vi "Read All Segments.vi"(8 "error in (no error)":errorcluster, 9 "Timeout (10000 ms)":u32=10000, 10 "Source (0: Channel 1)":u16(ring) items=["Channel 1", "Channel 2", "Channel 3", "Channel 4", "Memory 1", "Memory 2", "Memory 3", "Memory 4", "Function 1", "Function 2", "Function 3", "Function 4", "Function 5", "Function 6", "Function 7", "Function 8"], 11 "VISA resource name":refnum<visa-resource-name>) -> (0 "error out":errorcluster, 2 "Max Waveform":waveform(dbl)[](graph), 3 "VISA resource name out":refnum<visa-resource-name>)   [LabVIEW 2013, in "LeCroy Wave Series.lvlib"]
doc: "Returns the alls segments of waveform the oscilloscope acquired for the specified channel. The waveform is from an acquisition that you initiate prior to calling this VI.\n\nNote:\n\nSequence Acquisitions are not supported by WaveSurfer models."
uses:
  LeCroy Wave Series.lvlib
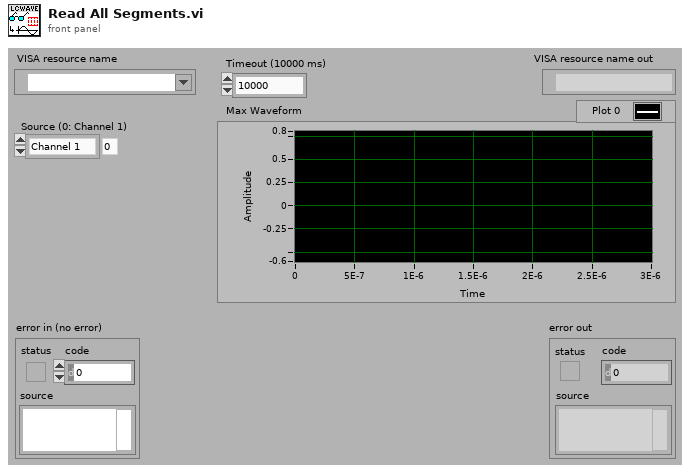
[diagram p1: front panel]
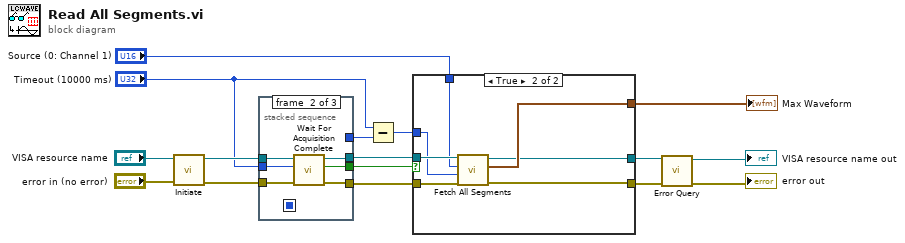
[diagram p0: block diagram]
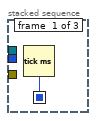
[diagram p2: hidden frame]
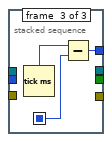
[diagram p3: hidden frame]
diagram:
  n1 = call "Initiate.vi"("error in (no error)"="error in (no error)", "VISA resource name"="VISA resource name") -> ("error out"=w11:errorcluster, "VISA resource name out"=w12:refnum<visa-resource-name>)  [unwired: 8 in]
  n2 = stacked-sequence {
    seq-local: [w17 _ _] -> [_ _ w25]
    tunnel: "Timeout (10000 ms)" -> [_ w23 _]
    tunnel: w12 -> [_ w21 _]
    tunnel: w11 -> [_ w19 _]
    tunnel: [_ w18 _] -> w9
    tunnel: [_ w20 _] -> w10
    tunnel: [_ _ w24] -> w7
    tunnel: [_ w22 _] -> w5
    frame #0 {
      n3 = Tick Count (ms)() -> (millisecond timer value=w17:u32)
    }
    frame #1 {
      n4 = call "Wait For Acquisition Complete.vi"("error in (no error)"=w19, "Timeout (10000 ms)"=w23, "VISA resource name"=w21) -> ("error out"=w18:errorcluster, "Complete"=w22:bool, "VISA resource name out"=w20:refnum<visa-resource-name>)  [unwired: 6 in]
    }
    frame #2 {
      n5 = Tick Count (ms)() -> (millisecond timer value=w26:u32)
      n6 = Subtract(x=w26, y=w25) -> (x-y=w24:u32)
    }
  }
  n7 = Subtract(x="Timeout (10000 ms)", y=w7) -> (x-y=w6:u32)
  n8 = case shown="True" w5 {
    tunnel: w10 -> [w28 w35]
    tunnel: w9 -> [w27 w34]
    tunnel: "Source (0: Channel 1)" -> [_ w33]
    tunnel: [_ w32] -> w13
    tunnel: [w28 w31] -> w4
    tunnel: [w27 w30] -> w2
    tunnel: w6 -> [_ w29]
    frame False {
    }
    frame True {
      n9 = call "Fetch All Segments.vi"("error in (no error)"=w34, "Timeout (10000 ms)"=w29, "Source (0: Channel 1)"=w33, "VISA resource name"=w35) -> ("error out"=w30:errorcluster, "Array"=w32:waveform(dbl)[], "VISA resource name out"=w31:refnum<visa-resource-name>)  [unwired: 5 in]
    }
  }
  "Max Waveform" <- w13
  n10 = call "Error Query.vi"("error in (no error)"=w2, "VISA resource name"=w4) -> ("error out"=→"error out":errorcluster, "VISA resource name out"=→"VISA resource name out":refnum<visa-resource-name>)  [unwired: 6 in, 2 out]
